vi "Version.vi"(0 "reference in":refnum<class "Driver_Template.lvclass">, 11 "error in (no error)":errorcluster) -> (4 "reference in":refnum<class "Driver_Template.lvclass">, 6 "Class":string, 8 "Version":string, 10 "Chain":string, 15 "error out":errorcluster)   [LabVIEW 2014]
uses:
  Driver_Template.lvclass
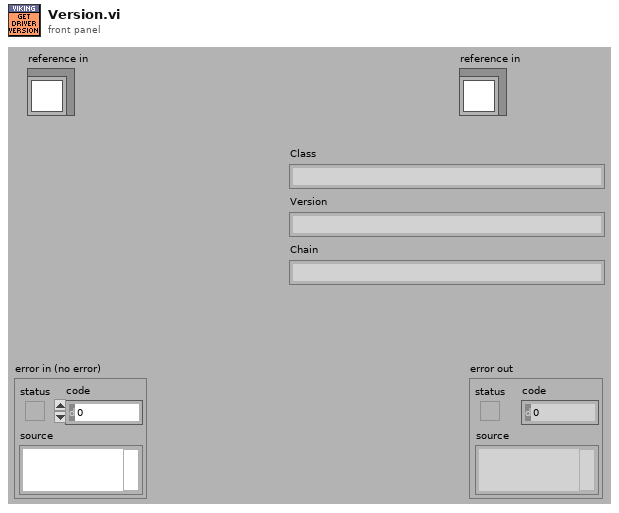
[diagram p1: front panel]
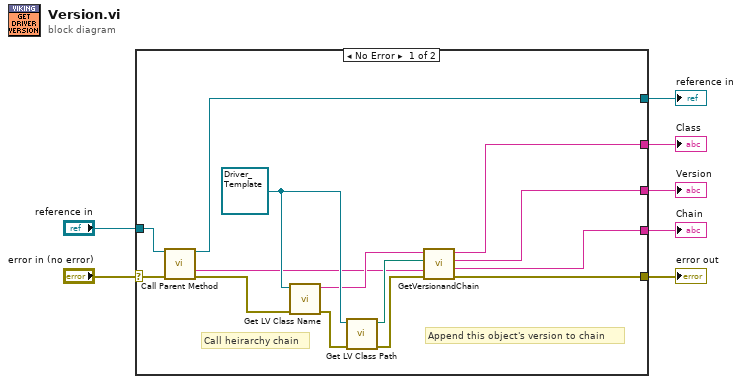
[diagram p0: block diagram]
diagram:
  n1 = case shown="No Error" "error in (no error)" {
    selector: "error in (no error)" -> [w19 w23]
    tunnel: [w14 w23] -> w6
    tunnel: [w20 w22] -> w4
    tunnel: "reference in" -> [w21 w22]
    tunnel: [w12 _] -> w3
    tunnel: [w13 _] -> w2
    tunnel: [w11 _] -> w1
    frame No Error {
      w16 = refnum<class "Driver_Template.lvclass"> refnum ("reference in")
      # "Call heirarchy chain"
      # "Append this object's version to chain"
      n2 = call-parent "Call Parent Method"("reference in"=w21, "error in (no error)"=w19) -> ("reference out"=w20:refnum<class "Driver_Template.lvclass">, "Chain"=w8:string, "error out"=w18:errorcluster)  [unwired: 9 in, 2 out]
      n3 = call <vilib>:"Get LV Class Name.vi"("error in (no error)"=w18, "object"=w16) -> ("error out"=w17:errorcluster, "class name"=w10:string)  [unwired: 8 in]
      n4 = call <vilib>:"Get LV Class Path.vi"("error in (no error)"=w17, "object"=w16) -> ("error out"=w15:errorcluster, "class path"=w9:path)  [unwired: 8 in]
      n5 = call "GetVersionandChain.vi"("error in (no error)"=w15, "Chain in"=w8, "class path in"=w9, "class name in"=w10) -> ("error out"=w14:errorcluster, "Chain out"=w13:string, "Version"=w12:string, "class name out"=w11:string)  [unwired: 4 in]
    }
    frame Error {
    }
  }
  "error out" <- w6
  "reference in" <- w4
  "Version" <- w3
  "Chain" <- w2
  "Class" <- w1
